vi "SIS.vi"   [LabVIEW 2017]
uses:
  <vilib>/Platform/TimedLoop/XDataNode/timing_clust.ctl
  <vilib>/Platform/TimedLoop/XDataNode/nitl_modes.ctl
  <vilib>/Platform/TimedLoop/XDataNode/wakeup.ctl
  <vilib>/Platform/TimedLoop/XDataNode/XDataNode.xnode
  <vilib>/Platform/TimedLoop/XDataNode/XDNodeRunTimeDep.lvlib
types:
  T1 = typedef "XDNodeRunTimeDep.lvlib/timing_clust.ctl" = cluster{"Expected End [f-1]":u64, "Actual End [f-1]":u64, "Finished Late? [f-1]":bool, "Expected End [i-1]":u64, "Actual End [i-1]":u64, "Finished Late? [i-1]":bool, "Expected Start [i]":u64, "Actual Start [i]":u64, "Expected Start [f]":u64, "Actual Start [f]":u64, "Source Name":string, "Structure Name":string, "Period":i64, "Deadline":i64, "Offset":i64, "Start":i64, "Priority":i32, "Timeout":i32, "Mode":T2, "Wakeup Reason":T3, "Error":errorcluster, "Source Type":string, "Secondary Source Type":string, "Global End Time":u64, "Global Start Time":u64, "Frame Duration":u64, "Iteration Duration":u64, "Assigned CPU":i32, "I/O Scan Engine Mode":u32}
  T2 = typedef "XDNodeRunTimeDep.lvlib/nitl_modes.ctl" = enum32{"No Change", "Process missed periods, maintain original phase", "Discard missed periods, maintain original phase", "Process missed periods, ignore original phase", "Discard missed periods, ignore original phase"}
  T3 = typedef "XDNodeRunTimeDep.lvlib/wakeup.ctl" = enum32{"Normal", "Aborted", "Asynchronous wakeup", "Timing source error", "Timed loop error", "Timeout"}
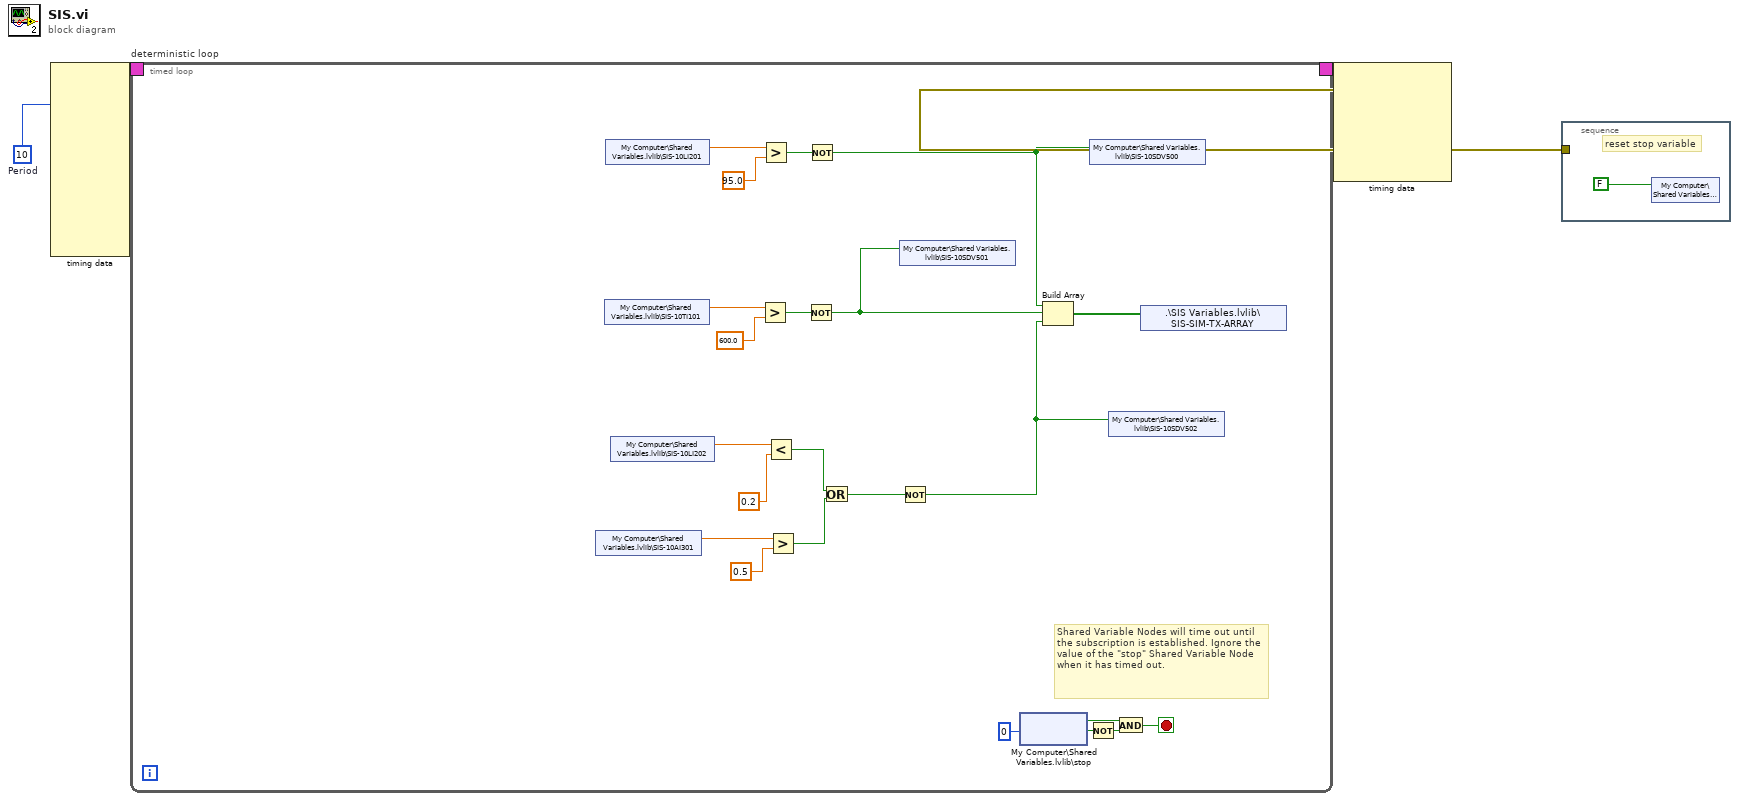
[diagram p0: block diagram]
diagram:
  w2 = i64 10  # Period
  n1 = node-c288 ("Input Node")(w2) -> (w4:T1)  [unwired: 9 in]
  n2 = timed-loop "deterministic loop" {
    timing: w4 -> [_]
    timing-out: [_] -> w3
    stop <- w26 stop-if-true
    # "Shared Variable Nodes will time out until the subscription is established. Ignore the value of the \"stop\" Shared Variable Node when it has timed out."
    n3 = shared-variable "My Computer\\Shared Variables.lvlib\\SIS-10AI301"() -> (w13:dbl)  [unwired: 1 in, 1 out]
    n4 = shared-variable "My Computer\\Shared Variables.lvlib\\SIS-10TI101"() -> (w16:dbl)  [unwired: 1 in, 1 out]
    n5 = shared-variable "My Computer\\Shared Variables.lvlib\\SIS-10LI201"() -> (w19:dbl)  [unwired: 1 in, 1 out]
    n6 = shared-variable "My Computer\\Shared Variables.lvlib\\SIS-10LI202"() -> (w15:dbl)  [unwired: 1 in, 1 out]
    n7 = Greater?(x=w16, y=600.0) -> (0:w17:bool)
    n8 = Greater?(x=w19, y=95.0) -> (0:w20:bool)
    n9 = Less?(x=w15, y=0.2) -> (x < y?=w12:bool)
    n10 = Greater?(x=w13, y=0.5) -> (0:w11:bool)
    n11 = Not(x=w17) -> (.not. x?=w6:bool)
    n12 = Not(x=w20) -> (.not. x?=w7:bool)
    n13 = Or(x=w12, y=w11) -> (x .or. y?=w10:bool)
    n14 = shared-variable "My Computer\\Shared Variables.lvlib\\SIS-10SDV501"(w6) -> ()  [unwired: 1 in, 1 out]
    n15 = Not(x=w10) -> (.not. x?=w5:bool)
    n16 = shared-variable "My Computer\\Shared Variables.lvlib\\stop"(0 ("ms timeout (0)")) -> (w23:bool, w24:bool)  [unwired: 1 in, 1 out]
    n17 = Build Array(w7, w6, w5) -> (w8:bool[])
    n18 = Not(x=w24) -> (.not. x?=w25:bool)
    n19 = shared-variable "My Computer\\Shared Variables.lvlib\\SIS-10SDV500"(w7) -> ()  [unwired: 1 in, 1 out]
    n20 = shared-variable "My Computer\\Shared Variables.lvlib\\SIS-10SDV502"(w5) -> ()  [unwired: 1 in, 1 out]
    n21 = And(x=w23, y=w25) -> (x .and. y?=w26:bool)
    n22 = shared-variable ".\\SIS Variables.lvlib\\SIS-SIM-TX-ARRAY"(w8) -> ()  [unwired: 1 in, 1 out]
  }
  n23 = node-c288 ("Output Node")(w3) -> (w1:errorcluster)  [unwired: 5 out]
  n24 = stacked-sequence {
    tunnel: w1 -> [_]
    frame #0 {
      # "reset stop variable"
      n25 = shared-variable "My Computer\\Shared Variables.lvlib\\stop"(FALSE) -> ()  [unwired: 1 in, 1 out]
    }
  }
